vi "ErrorHandling.loadCustomErrors.vi"(8 "error in (no error)":errorcluster, 11 "ErrorHandling in":refnum<data-value>) -> (0 "error out":errorcluster, 3 "ErrorHandling out":refnum<data-value>)   [LabVIEW 2016, in "ErrorHandling.lvclass"]
uses:
  ErrorHandling.lvclass
  ErrorHandling.lvclass/ErrorHandling.ctl
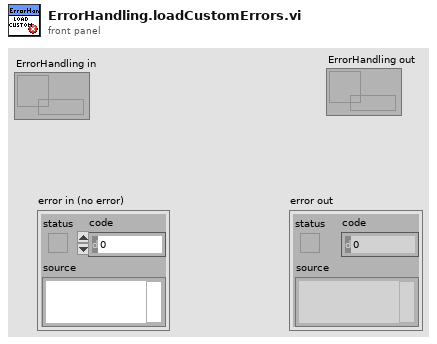
[diagram p1: front panel]
types:
  T1 = enum16{"open", "replace", "create", "open or create", "replace or create", "replace or create with confirmation"}
  T2 = cluster{errorcluster, "Action":enum16{"continue", "stop"}, string}
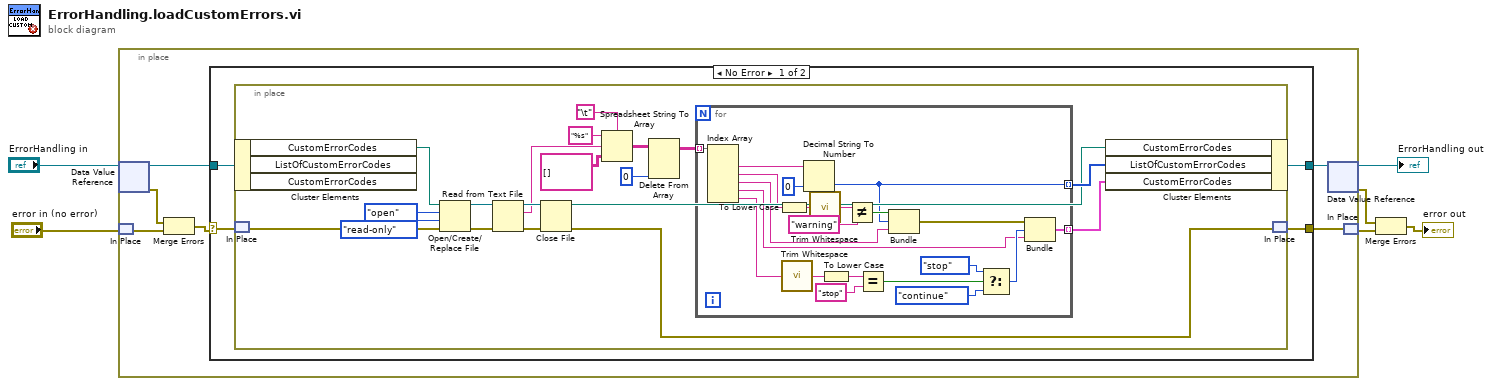
[diagram p0: block diagram]
diagram:
  n1 = in-place {
    n2 = in-place-dvr #1("ErrorHandling in") -> (w12:refnum<class "ErrorHandling.lvclass">, w7:errorcluster)
    n3 = in-place-match #2("error in (no error)") -> (w9:errorcluster)
    n4 = Merge Errors(w7, w9) -> (w10:errorcluster)
    n5 = case shown="No Error" w10 {
      selector: w10 -> [w14 w58]
      tunnel: [w13 w58] -> w8
      tunnel: [w15 w57] -> w11
      tunnel: w12 -> [w16 w57]
      frame No Error {
        n6 = in-place {
          n7 = in-place-cluster #3(w16) -> ("CustomErrorCodes"=w20:path)  [unwired: 2 out]
          n8 = in-place-match #4(w14) -> (w18:errorcluster)
          n9 = Open/Create/Replace File(file path (use dialog)=w20, error in=w18, operation (0:open)=T1."open", access (0:read/write)=enum16{"read/write", "read-only", "write-only"}."read-only") -> (refnum out=w31:refnum<file>, error out=w30:errorcluster)  [unwired: 2 in, 1 out]
          n10 = Read from Text File(file (use dialog)=w31, error in=w30) -> (refnum out=w32:refnum<file>, text=w29:string, error out=w33:errorcluster)  [unwired: 2 in, 1 out]
          n11 = Close File(refnum=w32, error in=w33) -> (path=w21:path, error out=w17:errorcluster)
          n12 = Spreadsheet String To Array(delimiter (Tab)="\t", format string="%s", spreadsheet string=w29, array type (2D Dbl)=string[][] []) -> (array=w25:string[][])
          n13 = Delete From Array(array=w25, index (row)=0) -> (array with subset deleted=w24:string[][])  [unwired: 2 in, 1 out]
          n14 = for {
            tunnel: w24 -> [w56] mode=indexing
            tunnel: [w44] -> w19 mode=indexing
            tunnel: [w38] -> w22 mode=indexing
            n15 = Index Array(array=w56) -> (element #1=w55:string, element #2=w54:string, element #3=w48:string, element #4=w36:string, element #5=w37:string)  [unwired: 5 in]
            n16 = To Lower Case(string=w54) -> (all lower case string=w52:string)
            n17 = call <vilib>:"Trim Whitespace.vi"("string"=w37) -> ("trimmed string"=w47:string)  [unwired: 1 in]
            n18 = Decimal String To Number(string=w55, default (0L)=0 ("default (0 I32)")) -> (number=w38:i32)  [unwired: 1 in, 1 out]
            n19 = call <vilib>:"Trim Whitespace.vi"("string"=w52) -> ("trimmed string"=w51:string)  [unwired: 1 in]
            n20 = To Lower Case(string=w47) -> (all lower case string=w46:string)
            n21 = Not Equal?(x=w51, y="warning") -> (x != y?=w49:bool)
            n22 = Equal?(x=w46, y="stop") -> (x = y?=w41:bool)
            n23 = Bundle(w49, w38, w48) -> (w45:errorcluster)  [unwired: 1 in]
            n24 = Select(t=enum16{"continue", "stop"}."stop" ("Action"), s=w41, f=enum16{"continue", "stop"}."continue" ("Action")) -> (s? t:f=w40:enum16{"continue", "stop"})
            n25 = Bundle(w45, "Action"=w40, w36) -> (w44:T2)  [unwired: 1 in]
          }
          n26 = in-place-cluster #3("CustomErrorCodes"=w21, "ListOfCustomErrorCodes"=w22, "CustomErrorCodes"=w19) -> (w15:refnum<class "ErrorHandling.lvclass">)
          n27 = in-place-match #4(w17) -> (w13:errorcluster)
        }
      }
      frame Error {
      }
    }
    n28 = in-place-dvr #1(w11) -> (→"ErrorHandling out":refnum<data-value>, w4:errorcluster)
    n29 = in-place-match #2(w8) -> (w1:errorcluster)
  }
  n30 = Merge Errors(w4, w1) -> (→"error out":errorcluster)
